vi "Qualify Library Icon Core.vi"(0 "VI Reference":refnum<vi>, 11 "error in":errorcluster) -> (3 "Class?":bool, 4 "Good Library Icon":bool, 6 "Maximum Number of Rows":i32, 8 "Library Path":path, 10 "Number of Rows in Icon":i32, 14 "Icon Image":picture, 15 "error out":errorcluster)   [LabVIEW 2020, in "Text-Based VI Icon.lvlib"]
uses:
  <vilib>/LabVIEW Icon API/Set Text Icon/Text-Based VI Icon.lvlib
panel:
  out "Left and Right Good (for Debugging)":bool
  out "Top and Bottom Good (for Debugging)":bool
  out "Good Frame Color (for Debugging)":bool
  out "Supported Size or Shape (for Debugging)":bool
  out "Last True Mask + 1 (for Debugging)":i32
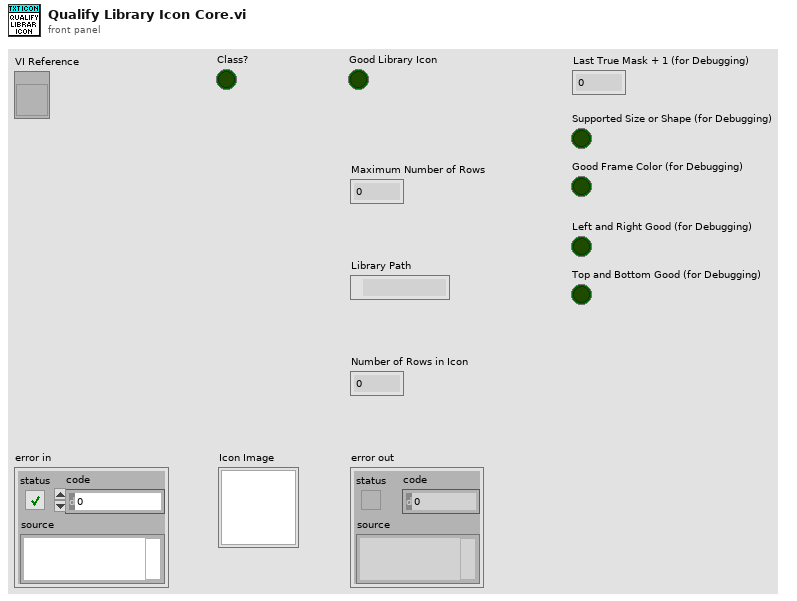
[diagram p1: front panel]
types:
  T1 = typedef "imagedata.ctl" = cluster{"image type":i32, "image depth":i32, "image":u8[], "mask":u8[], "colors":u32[], "Rectangle":cluster{"left":i16, "top":i16, "right":i16, "bottom":i16}}
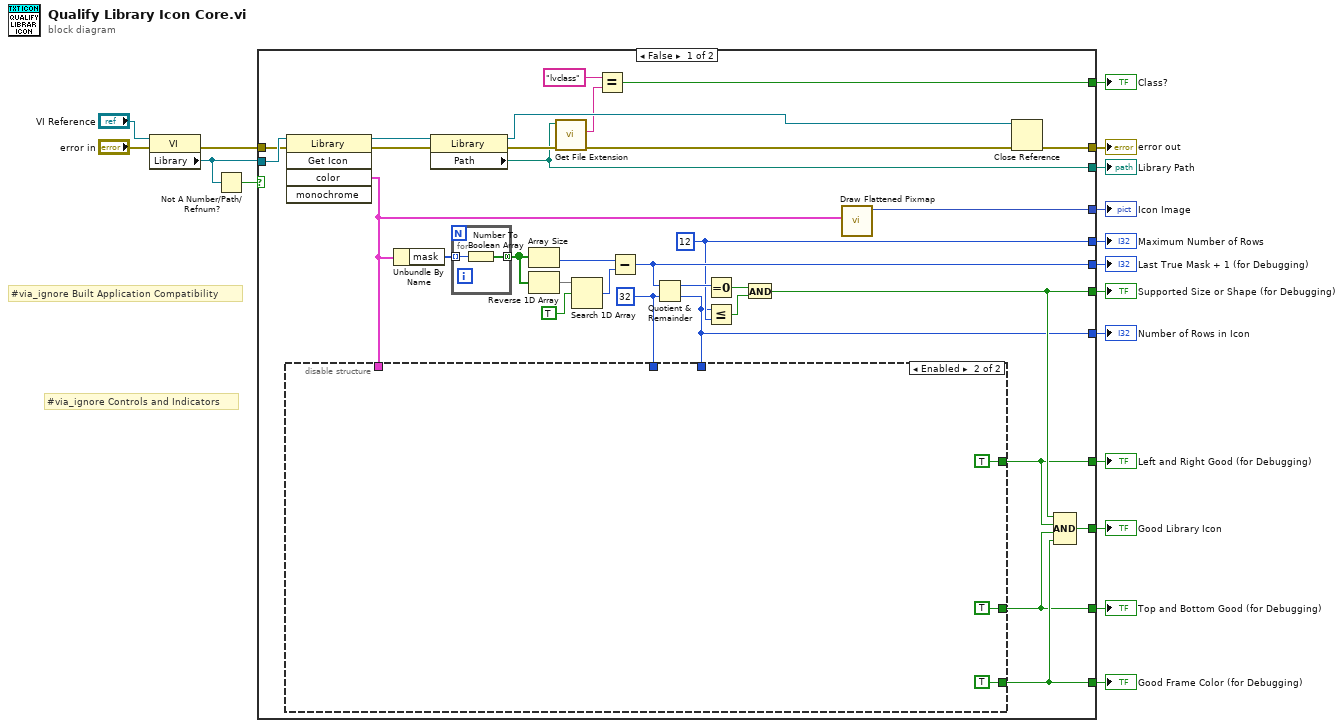
[diagram p0: block diagram]
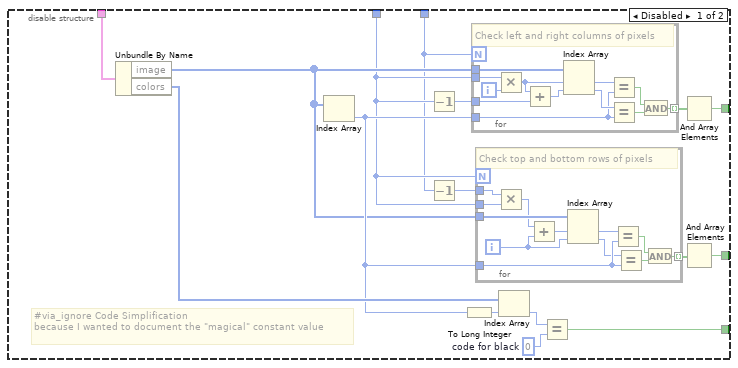
[diagram p2: hidden frame]
diagram:
  # "#via_ignore Built Application Compatibility"
  # "#via_ignore Controls and Indicators"
  n1 = property class="VI"(reference="VI Reference", error in="error in") -> (error out=w15:errorcluster, "Library"=w16:refnum<vi>)  [unwired: 1 out]
  n2 = Not A Number/Path/Refnum?(number/path/refnum=w16) -> (NaN/Path/Refnum?=w17:bool)
  n3 = case shown="False" w17 {
    tunnel: w16 -> [w49 _]
    tunnel: w15 -> [w48 w95]
    tunnel: [w27 w95] -> w14
    tunnel: [w38 _] -> w13
    tunnel: [w35 _] -> w12
    tunnel: [w33 _] -> w11
    tunnel: [w32 _] -> w10
    tunnel: [w34 _] -> w9
    tunnel: [w36 _] -> w8
    tunnel: [w31 _] -> w7
    tunnel: [w20 _] -> w6
    tunnel: [w28 _] -> w3
    tunnel: [w21 _] -> w2
    tunnel: [w18 _] -> w1
    frame False {
      w28 = 12 ("y")
      w37 = 32 ("y")
      n4 = invoke class="Library" method="Get Icon"(reference=w49, error in=w48) -> (reference out=w30:refnum<vi>, error out=w29:errorcluster, "color"=w19:T1)  [unwired: 3 in, 2 out]
      n5 = Unbundle By Name(w19) -> ("mask"=w44:u8[])
      n6 = property class="Library"(reference=w30, error in=w29) -> (reference out=w26:refnum<vi>, error out=w25:errorcluster, "Path"=w20:path)
      n7 = for {
        tunnel: w44 -> [w94] mode=indexing
        tunnel: [w93] -> w41 mode=concatenating
        n8 = Number To Boolean Array(number=w94) -> (Boolean array=w93:bool[])
      }
      n9 = Array Size(array=w41) -> (size(s)=w40:i32)
      n10 = Reverse 1D Array(array=w41) -> (reversed array=w43:bool[])
      n11 = call <vilib>:"Get File Extension.vi"("error in (no error)"=w25, "file"=w20) -> ("error out"=w24:errorcluster, "lowercase file extension"=w23:string)  [unwired: 5 in, 3 out]
      n12 = Search 1D Array(1D array=w43, element=TRUE) -> (index of element=w39:i32)  [unwired: 1 in]
      n13 = Equal?(x="lvclass", y=w23) -> (x = y?=w21:bool)
      n14 = Subtract(x=w40, y=w39) -> (x-y=w38:i32)
      n15 = Quotient & Remainder(x=w38, y=w37) -> (x-y*floor(x/y)=w47:i32, floor(x/y)=w18:i32)
      n16 = disable-structure shown="Enabled" {
        disable-tunnel: w37 -> [w55 _]
        disable-tunnel: [w54 TRUE] -> w34
        disable-tunnel: [w53 TRUE] -> w33
        disable-tunnel: [w52 TRUE] -> w32
        disable-tunnel: w19 -> [w51 _]
        disable-tunnel: w18 -> [w50 _]
        frame Disabled {
          w64 = u32 0  # code for black
          # "#via_ignore Code Simplification\nbecause I wanted to document the \"magical\" constant value"
          n17 = Unbundle By Name(w51) -> ("image"=w59:u8[], "colors"=w65:u32[])
          n18 = Index Array(array=w59) -> (element=w60:u8)  [unwired: 1 in]
          n19 = Decrement(x=w55) -> (x-1=w57:i32)
          n20 = Decrement(x=w50) -> (x-1=w61:i32)
          n21 = To Long Integer(number=w60) -> (32bit integer=w63:i32)
          n22 = for {
            N: w50 -> [_]
            tunnel: w60 -> [w79]
            tunnel: [w87] -> w58 mode=indexing
            tunnel: w57 -> [w85]
            tunnel: w59 -> [w83]
            tunnel: w55 -> [w81]
            i -> [w86]
            # "Check left and right columns of pixels"
            n23 = Multiply(x=w81, y=w86) -> (x*y=w78:i32)
            n24 = Add(x=w78, y=w85) -> (x+y=w80:i32)
            n25 = Index Array(array=w83, index #1=w78, index #2=w80) -> (element #1=w82:u8, element #2=w84:u8)
            n26 = Equal?(x=w82, y=w79) -> (x = y?=w89:bool)
            n27 = Equal?(x=w84, y=w79) -> (x = y?=w88:bool)
            n28 = And(x=w89, y=w88) -> (x .and. y?=w87:bool)
          }
          n29 = for {
            N: w55 -> [_]
            tunnel: w59 -> [w77]
            tunnel: w61 -> [w76]
            tunnel: w60 -> [w71]
            tunnel: [w67] -> w62 mode=indexing
            tunnel: w55 -> [w66]
            i -> [w73]
            # "Check top and bottom rows of pixels"
            n30 = Multiply(x=w76, y=w66) -> (x*y=w75:i32)
            n31 = Add(x=w75, y=w73) -> (x+y=w74:i32)
            n32 = Index Array(array=w77, index #1=w74, index #2=w73) -> (element #1=w72:u8, element #2=w70:u8)
            n33 = Equal?(x=w72, y=w71) -> (x = y?=w69:bool)
            n34 = Equal?(x=w70, y=w71) -> (x = y?=w68:bool)
            n35 = And(x=w69, y=w68) -> (x .and. y?=w67:bool)
          }
          n36 = Index Array(array=w65, index=w63) -> (element=w56:u32)
          n37 = Equal?(x=w56, y=w64) -> (x = y?=w53:bool)
          n38 = And Array Elements(Boolean array=w58) -> (logical AND=w54:bool)
          n39 = And Array Elements(Boolean array=w62) -> (logical AND=w52:bool)
        }
        frame Enabled {
        }
      }
      n40 = Equal To 0?(x=w47) -> (x = 0?=w46:bool)
      n41 = Less Or Equal?(x=w18, y=w28) -> (x <= y?=w45:bool)
      n42 = And(x=w46, y=w45) -> (x .and. y?=w35:bool)
      n43 = call <vilib>:"Draw Flattened Pixmap.vi"("image data"=w19) -> ("new picture"=w36:picture)  [unwired: 8 in]
      n44 = Close Reference(reference=w26, error in (no error)=w24) -> (error out=w27:errorcluster)
      n45 = Compound Arithmetic op=AND(w35, w34, w32, w33) -> (w31:bool)
    }
    frame True {
    }
  }
  "error out" <- w14
  "Last True Mask + 1 (for Debugging)" <- w13
  "Supported Size or Shape (for Debugging)" <- w12
  "Good Frame Color (for Debugging)" <- w11
  "Top and Bottom Good (for Debugging)" <- w10
  "Left and Right Good (for Debugging)" <- w9
  "Icon Image" <- w8
  "Good Library Icon" <- w7
  "Library Path" <- w6
  "Maximum Number of Rows" <- w3
  "Class?" <- w2
  "Number of Rows in Icon" <- w1
